vi "Get Test Modes.vi"(11 "First Row":string[](array[string])) -> (3 "Test Modes Out":string[](array[string]))   [LabVIEW 2018, in "Test Number and Bin Generator.lvlib" / "Test Number and Bin Generator.lvclass"]
uses:
  Test Number and Bin Generator.lvclass
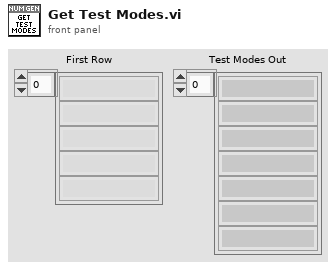
[diagram p1: front panel]
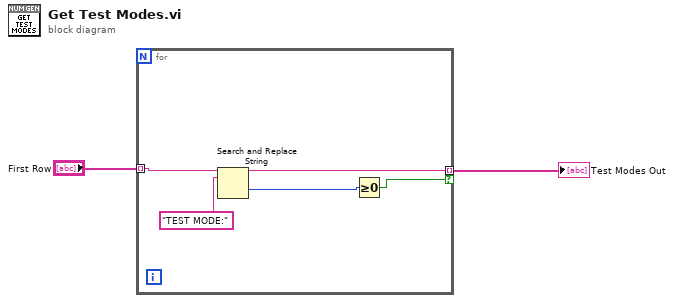
[diagram p0: block diagram]
diagram:
  n1 = for {
    tunnel: "First Row" -> [w7] mode=indexing
    tunnel: [w5] -> w1 mode=indexing if=w3
    n2 = Search and Replace String(input string=w7, search string="TEST MODE:" ("format string")) -> (result string=w5:string, offset past replacement=w4:i32)  [unwired: 6 in, 2 out]
    n3 = Greater Or Equal To 0?(x=w4) -> (x >= 0?=w3:bool)
  }
  "Test Modes Out" <- w1
